vi "createCamera.vi"(8 "error in (no error)":errorcluster, 9 "machine name":string, 10 "Camera":string, 11 "NetworkPixelfly in":refnum<class "NetworkPixelfly.lvclass">) -> (0 "error out":errorcluster, 3 "NetworkPixelfly out":refnum<class "NetworkPixelfly.lvclass">)   [LabVIEW 2009, in "Hardware.lvlib" / "HWControllers.lvlib" / "NetworkPixelfly.lvclass"]
uses:
  NetworkPixelfly.lvclass
  Channels/Camera/PixelflySA/PixelflySA.lvclass
  Tools/Filing/FileSystem/FileSystem.lvclass
  NetworkPixelfly.lvclass/NetworkPixelfly.ctl
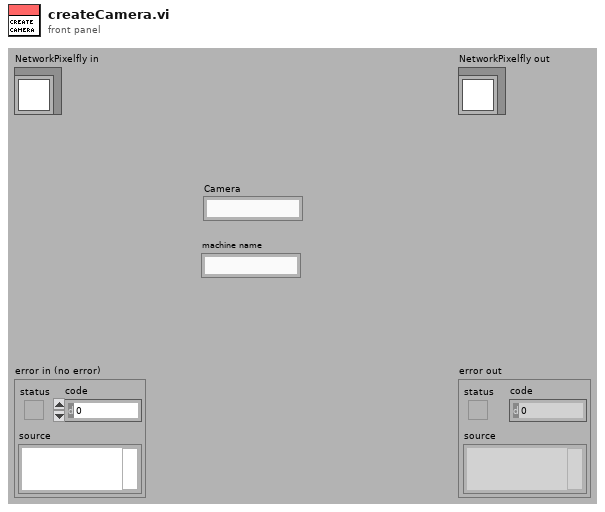
[diagram p1: front panel]
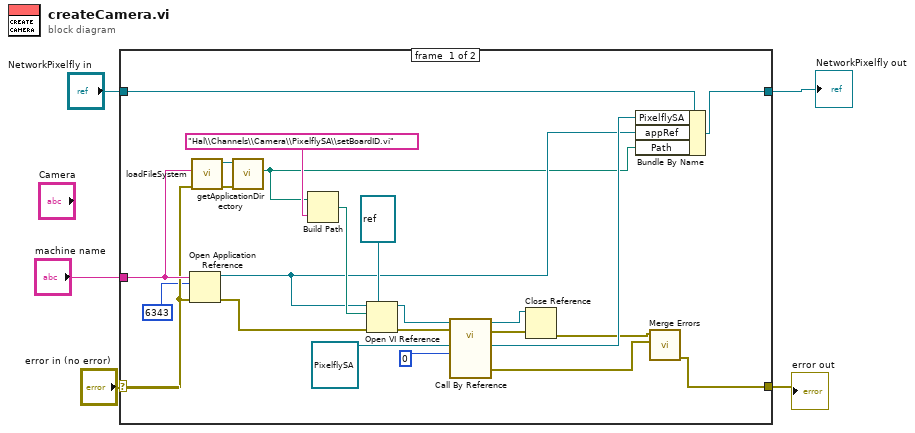
[diagram p0: block diagram]
diagram:
  n1 = case shown="No Error" "error in (no error)" {
    selector: "error in (no error)" -> [w22 w29]
    tunnel: [w15 w30] -> w5
    tunnel: "NetworkPixelfly in" -> [w16 w30]
    tunnel: [w12 w29] -> w2
    tunnel: "machine name" -> [w23 _]
    frame #0 {
      n2 = Open Application Reference(8:w22, 10:6343, 11:w23) -> (0:w24:errorcluster, 3:w8:refnum<vi>)  [unwired: 1 in]
      n3 = call "loadFileSystem.vi"("error in (no error)"=w22, "computer name"=w23) -> ("error out"=w27:errorcluster, "FileSystem out"=w28:refnum<class "FileSystem.lvclass">)  [unwired: 8 in]
      n4 = call-dynamic "getApplicationDirectory.vi"("error in (no error)"=w27, "FileSystem.lvclass in"=w28) -> ("ApplicationDirectory"=w7:path)  [unwired: 7 in, 2 out]
      n5 = Build Path(base path=w7, name or relative path="Hal\\Channels\\Camera\\PixelflySA\\setBoardID.vi") -> (appended path=w25:path)
      n6 = Open VI Reference(type specifier VI Refnum (for type only)=refnum<vi> refnum, application reference (local)=w8, vi path=w25, error in (no error)=w24) -> (vi reference=w21:refnum<vi>, error out=w17:errorcluster)  [unwired: 2 in]
      n7 = call-by-ref "?"(reference=w21, error in=w17, "boardID"=0, "Pixelfly in"=refnum<class "PixelflySA.lvclass"> refnum ("PixelflySA.lvclass")) -> (reference out=w11:refnum<vi>, error out=w10:errorcluster, 0:"error out"=w13:errorcluster, "Pixelfly out"=w14:refnum<class "PixelflySA.lvclass">)  [unwired: 8 in]
      n8 = Close Reference(reference=w11, error in (no error)=w10) -> (error out=w9:errorcluster)
      n9 = Bundle By Name(cluster=w16, "PixelflySA"=w14, "appRef"=w8, "Path"=w7) -> (w15:refnum<class "NetworkPixelfly.lvclass">)
      n10 = call <vilib>:"Merge Errors.vi"("error in 2 (no error)"=w13, "error in 1 (no error)"=w9) -> ("error out"=w12:errorcluster)  [unwired: 5 in]
    }
    frame #1 {
    }
  }
  "error out" <- w2
  "NetworkPixelfly out" <- w5
